vi "Start.vi"(8 "error in (no error)":errorcluster, 10 "Message in":refnum<class "StartMessage.lvclass">, 11 "BMC in":refnum<class "BMC.lvclass">) -> (0 "error out":errorcluster, 3 "BMC out":refnum<class "BMC.lvclass">)   [LabVIEW 2012, in "BMC.lvclass"]
doc: "This member function is called when the statemachine in the run.vi receives an 'start' command. It relays the message to all observers of the component.\n\nOverride this member function in your derived class if you need additional start functionality (but don't forget to call the parent method)."
uses:
  BMC.lvclass
  Murmex/LabVIEW/Murmex/Murmex/Murmex.lvclass
  Murmex/LabVIEW/Murmex/StartMessage/StartMessage.lvclass
panel:
  # "This member function is called when the statemachine in the run.vi receives an 'start' command. It relays the message to all observers of the component.\n\nOverride this member function in your derived class if you need additional start functionality (but don't forget to call the parent method)."
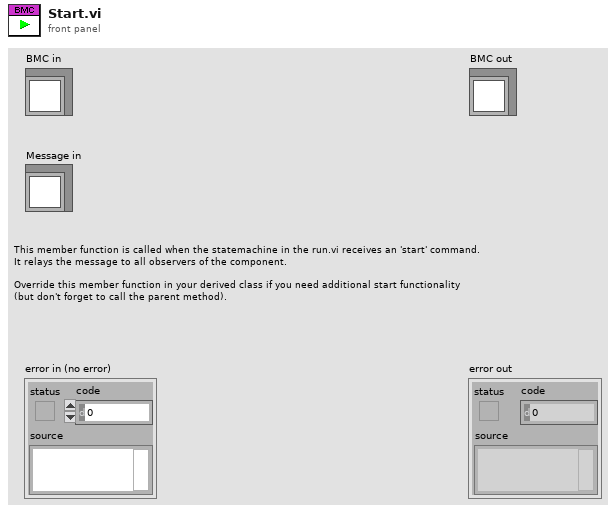
[diagram p1: front panel]
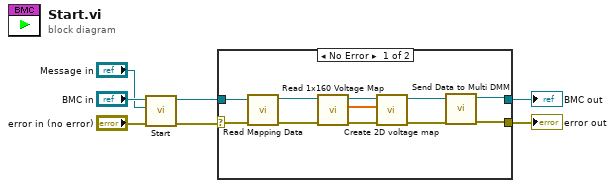
[diagram p0: block diagram]
diagram:
  n1 = call-parent "Start.vi"("error in (no error)"="error in (no error)", "Message in"="Message in", "Murmex in"="BMC in") -> ("error out"=w5:errorcluster, "Murmex out"=w2:refnum<class "BMC.lvclass">)  [unwired: 7 in]
  n2 = case shown="No Error" w5 {
    selector: w5 -> [w18 w19]
    tunnel: [w9 w19] -> w4
    tunnel: [w8 w20] -> w3
    tunnel: w2 -> [w17 w20]
    frame No Error {
      n3 = call-dynamic "Read Mapping Data.vi"("error in (no error)"=w18, "BMC in"=w17) -> ("error out"=w15:errorcluster, "BMC out"=w13:refnum<class "BMC.lvclass">)  [unwired: 7 in, 1 out]
      n4 = call-dynamic "Read 1x160 Voltage Map.vi"("error in (no error)"=w15, "BMC in"=w13) -> ("error out"=w14:errorcluster, "1x160  Voltage Map"=w16:dbl[], "BMC out"=w12:refnum<class "BMC.lvclass">)  [unwired: 7 in]
      n5 = call-dynamic "Create 2D voltage map.vi"("error in (no error)"=w14, "1x160  Voltage Map"=w16, "BMC in"=w12) -> ("error out"=w11:errorcluster, "BMC out"=w10:refnum<class "BMC.lvclass">)  [unwired: 6 in, 1 out]
      n6 = call-dynamic "Send Data to Multi DMM.vi"("error in (no error)"=w11, "BMC in"=w10) -> ("error out"=w9:errorcluster, "BMC out"=w8:refnum<class "BMC.lvclass">)  [unwired: 8 in]
    }
    frame Error {
    }
  }
  "error out" <- w4
  "BMC out" <- w3
